vi "CrossVertecies.vi"(5 "Cross X dimension\n(cross is square)":dbl) -> (2 "Combined":T2)   [LabVIEW 2014]
uses:
  Slicer/LVslicer/Slice/TypeDefs/Point2DwSlope.ctl
panel:
  in  "Beam Width":dbl
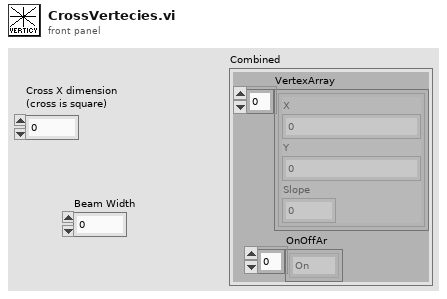
[diagram p1: front panel]
types:
  T1 = typedef "Point2DwSlope.ctl" = cluster{"X":sgl, "Y":sgl, "Slope":dbl}
  T2 = cluster{"VertexArray":T1[], "OnOffAr":enum16{"On", "Off"}[]}
  T3 = cluster{"Cross X dimension\n(cross is square)":dbl, dbl, dbl}
  T4 = cluster{dbl, "Cross X dimension\n(cross is square)":dbl, dbl}
  T5 = cluster{"Cross X dimension\n(cross is square)":dbl, "Cross X dimension\n(cross is square)":dbl, dbl}
  T6 = cluster{"Cross X dimension\n(cross is square)":dbl, "Cross X dimension\n(cross is square)":dbl, dbl}[]
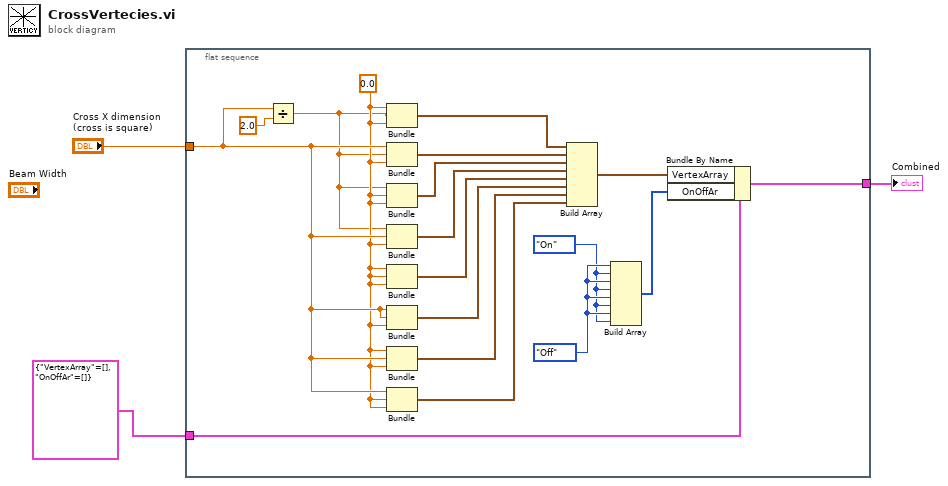
[diagram p0: block diagram]
diagram:
  n1 = flat-sequence {
    tunnel: T2 {"VertexArray"=[], "OnOffAr"=[]} ("Combined") -> [w9]
    tunnel: "Cross X dimension\n(cross is square)" -> [w20]
    tunnel: [w6] -> w1
    frame #0 {
      w4 = enum16{"On", "Off"}."On"
      w5 = enum16{"On", "Off"}."Off"
      w19 = 0.0
      n2 = Divide(x=w20, y=2.0) -> (x/y=w18:dbl)
      n3 = Bundle(w19, w18, w19) -> (w17:cluster{dbl, dbl, dbl})  [unwired: 1 in]
      n4 = Bundle("Cross X dimension\n(cross is square)"=w20, w18, w19) -> (w16:T3)  [unwired: 1 in]
      n5 = Bundle(w18, w19, w19) -> (w15:cluster{dbl, dbl, dbl})  [unwired: 1 in]
      n6 = Bundle(w18, "Cross X dimension\n(cross is square)"=w20, w19) -> (w14:T4)  [unwired: 1 in]
      n7 = Bundle(w19, w19, w19) -> (w13:cluster{dbl, dbl, dbl})  [unwired: 1 in]
      n8 = Bundle("Cross X dimension\n(cross is square)"=w20, "Cross X dimension\n(cross is square)"=w20, w19) -> (w12:T5)  [unwired: 1 in]
      n9 = Bundle(w19, "Cross X dimension\n(cross is square)"=w20, w19) -> (w11:T4)  [unwired: 1 in]
      n10 = Bundle("Cross X dimension\n(cross is square)"=w20, w19, w19) -> (w10:T3)  [unwired: 1 in]
      n11 = Build Array(w17, w16, w15, w14, w13, w12, w11, w10) -> (w7:T6)
      n12 = Build Array(w5, w4, w5, w4, w5, w4, w5, w4) -> (w8:enum16{"On", "Off"}[])
      n13 = Bundle By Name(cluster=w9, "VertexArray"=w7, "OnOffAr"=w8) -> (w6:T2)
    }
  }
  "Combined" <- w1
